vi "ECC read.vi"(9 "Address":dbl, 11 "Parameter code":dbl) -> (2 "Data array":dbl[](array[numeric]))   [LabVIEW 2010, in "Yudian AI508.lvlib"]
uses:
  <instrlib>/Yudian AI508/Yudian AI508.lvlib
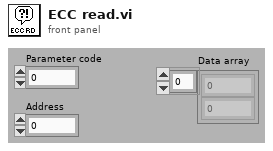
[diagram p1: front panel]
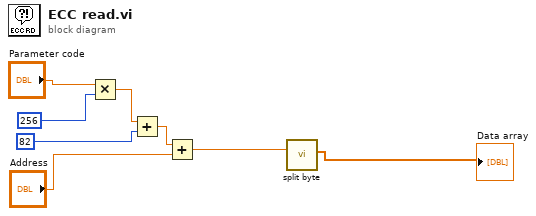
[diagram p0: block diagram]
diagram:
  n1 = Multiply(x="Parameter code", y=256) -> (x*y=w6:dbl)
  n2 = Add(x=w6, y=82) -> (x+y=w4:dbl)
  n3 = Add(x=w4, y="Address") -> (x+y=w2:dbl)
  n4 = call <instrlib>:"split byte.vi"("Value"=w2) -> ("Array"=→"Data array":dbl[])  [unwired: 10 in]
